vi "WT333.vi"(7 "simulazione":bool, 8 "error in (no error)":errorcluster, 11 "Queue Name":string="WT1600_Q") -> (0 "error out":errorcluster, 2 "Stopped":bool)   [LabVIEW 2019]
uses:
  TypeDef/MISURE WT.ctl
  TypeDef/DEVICE NAME.ctl
  <vilib>/Utility/file.llb/Read From Spreadsheet File (string).vi
  <vilib>/Utility/file.llb/Read Delimited Spreadsheet (string).vi
  <instrlib>/Yokogawa WT300 Series/Public/Data/Read Measurement (Normal).vi
  <instrlib>/Yokogawa WT300 Series/Yokogawa WT300 Series.lvlib
panel:
  out "length":i32
  out "read buffer 2":string
  out "Is Remote?":bool
  out "Is lockout?":bool
  in  "IS  REMOTE?":bool
  out "read buffer":string
  in  "IS LOCKOUT ?":bool
  in  "DIRETTO WT":bool
  in  "LEM 300":bool
  in  "LEM 1000":bool
  in  "LEM GENERICO":bool
  in  "write buffer":string=":INP:CURR:AUTO OFF;:INP:CURR:RANG EXT,1.0;"
  in  "CT Ratio (1.000)":dbl=0.2 format="%#_13g"
  out "Function":string[](array[string])
  out "WT330 Configuration":string[][](array[string])
  out "VISA resource name":refnum<visa-resource-name>
  in  "CONFIGURE":bool
  in  "SCELTA BANCO 2":bool
  out "Iteration":i32
  out "Measure":dbl[](array[numeric])
  out "MISURE WT":T1
  out "STATO":string
  out "LOOP TIME (ms)":u32
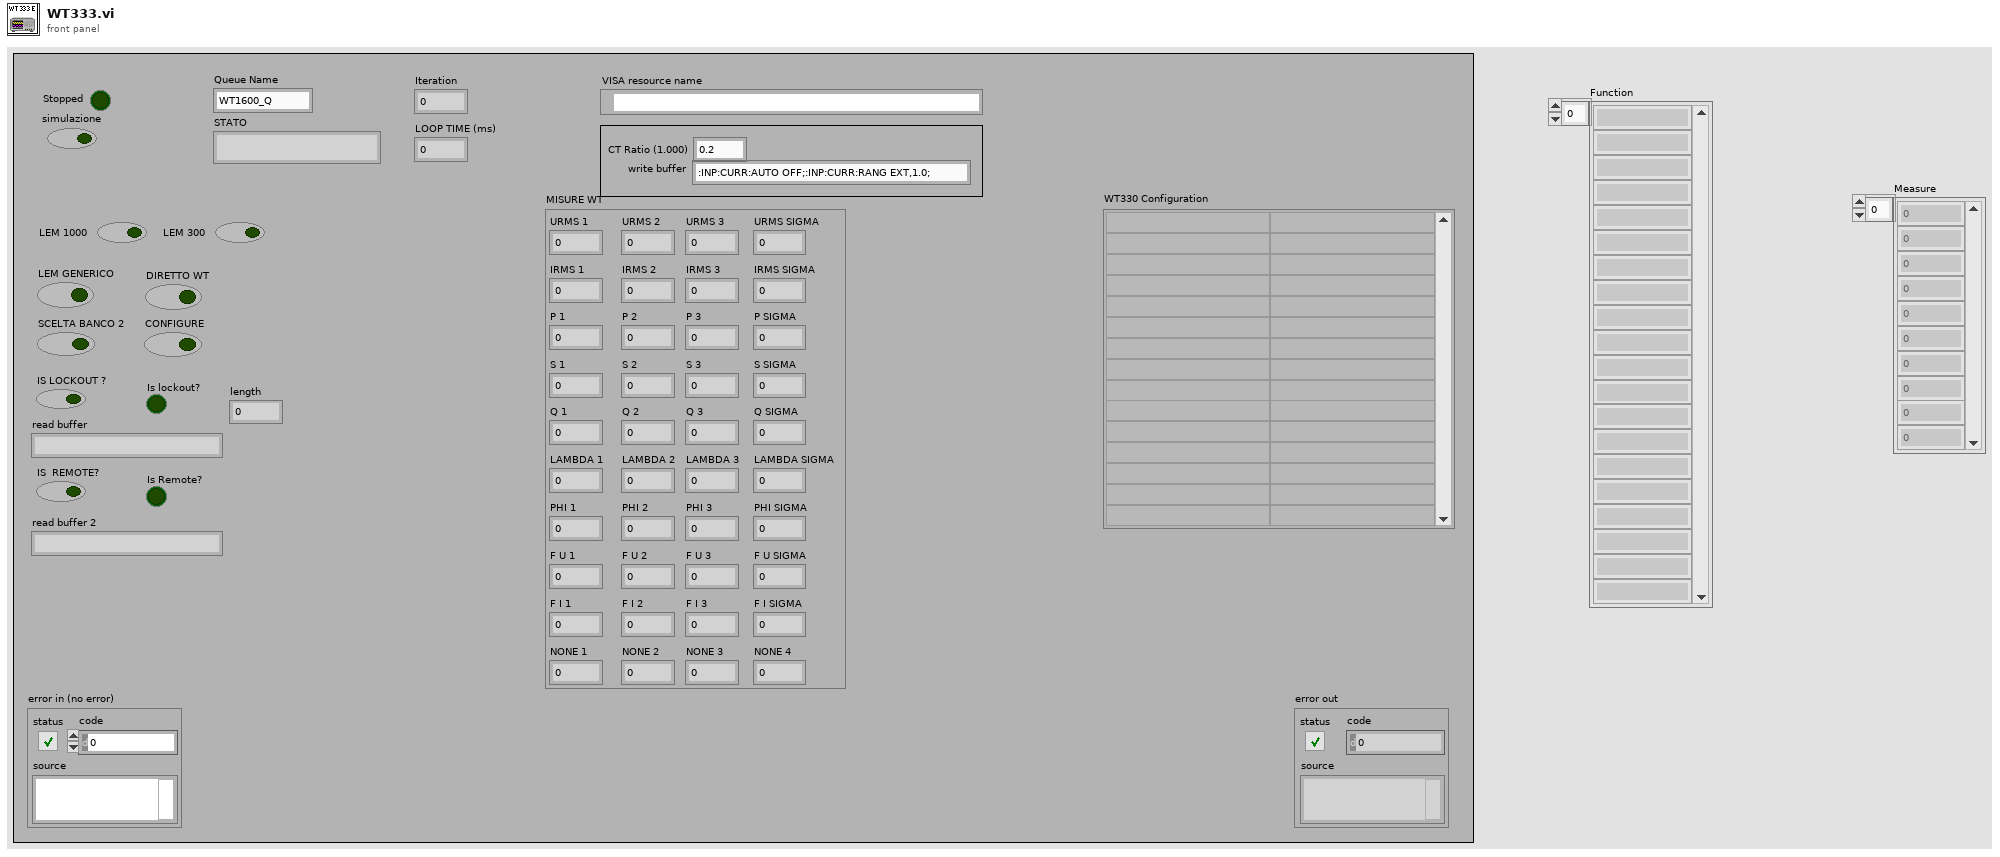
[diagram p1: front panel]
types:
  T1 = typedef "MISURE WT.ctl" = cluster{"URMS 1":dbl, "IRMS 1":dbl, "P 1":dbl, "S 1":dbl, "Q 1":dbl, "LAMBDA 1":dbl, "PHI 1":dbl, "F U 1":dbl, "F I 1":dbl, "NONE 1":dbl, "URMS 2":dbl, "IRMS 2":dbl, "P 2":dbl, "S 2":dbl, "Q 2":dbl, "LAMBDA 2":dbl, "PHI 2":dbl, "F U 2":dbl, "F I 2":dbl, "NONE 2":dbl, "URMS 3":dbl, "IRMS 3":dbl, "P 3":dbl, "S 3":dbl, "Q 3":dbl, "LAMBDA 3":dbl, "PHI 3":dbl, "F U 3":dbl, "F I 3":dbl, "NONE 3":dbl, "URMS SIGMA":dbl, "IRMS SIGMA":dbl, "P SIGMA":dbl, "S SIGMA":dbl, "Q SIGMA":dbl, "LAMBDA SIGMA":dbl, "PHI SIGMA":dbl, "F U SIGMA":dbl, "F I SIGMA":dbl, "NONE 4":dbl}
  T2 = typedef "DEVICE NAME.ctl" = enum16{"WATTMETRO", "APLUS", "PLC BANCO 1", "PLC RACK", "PLC BANCO 2", "PS", "NI cDAQ", "RESISTOMAT"}
  T3 = cluster{"Array of elements":cluster{"String":string, "variant":variant}[], "Single element":cluster{"String":string, "variant":variant}, "enque at\nopposite end (F)":bool, "no replications (F)":bool}
  T4 = cluster{"Measurement[0]":dbl, "Measurement[1]":dbl, "Measurement[2]":dbl, "Measurement[3]":dbl, "Measurement[4]":dbl, "Measurement[5]":dbl, "Measurement[6]":dbl, "Measurement[7]":dbl, "Measurement[8]":dbl, "Measurement[9]":dbl, "Measurement[10]":dbl, "Measurement[11]":dbl, "Measurement[12]":dbl, "Measurement[13]":dbl, "Measurement[14]":dbl, "Measurement[15]":dbl, "Measurement[16]":dbl, "Measurement[17]":dbl, "Measurement[18]":dbl, "Measurement[19]":dbl, "Measurement[20]":dbl, "Measurement[21]":dbl, "Measurement[22]":dbl, "Measurement[23]":dbl, "Measurement[24]":dbl, "Measurement[25]":dbl, "Measurement[26]":dbl, "Measurement[27]":dbl, "Measurement[28]":dbl, "Measurement[29]":dbl, "Measurement[30]":dbl, "Measurement[31]":dbl, "Measurement[32]":dbl, "Measurement[33]":dbl, "Measurement[34]":dbl, "Measurement[35]":dbl, "Measurement[36]":dbl, "Measurement[37]":dbl, "Measurement[38]":dbl, "Measurement[39]":dbl}
  T5 = enum32{"Invalid", "Standard", "Closed", "Hidden", "Minimized", "Maximized"}
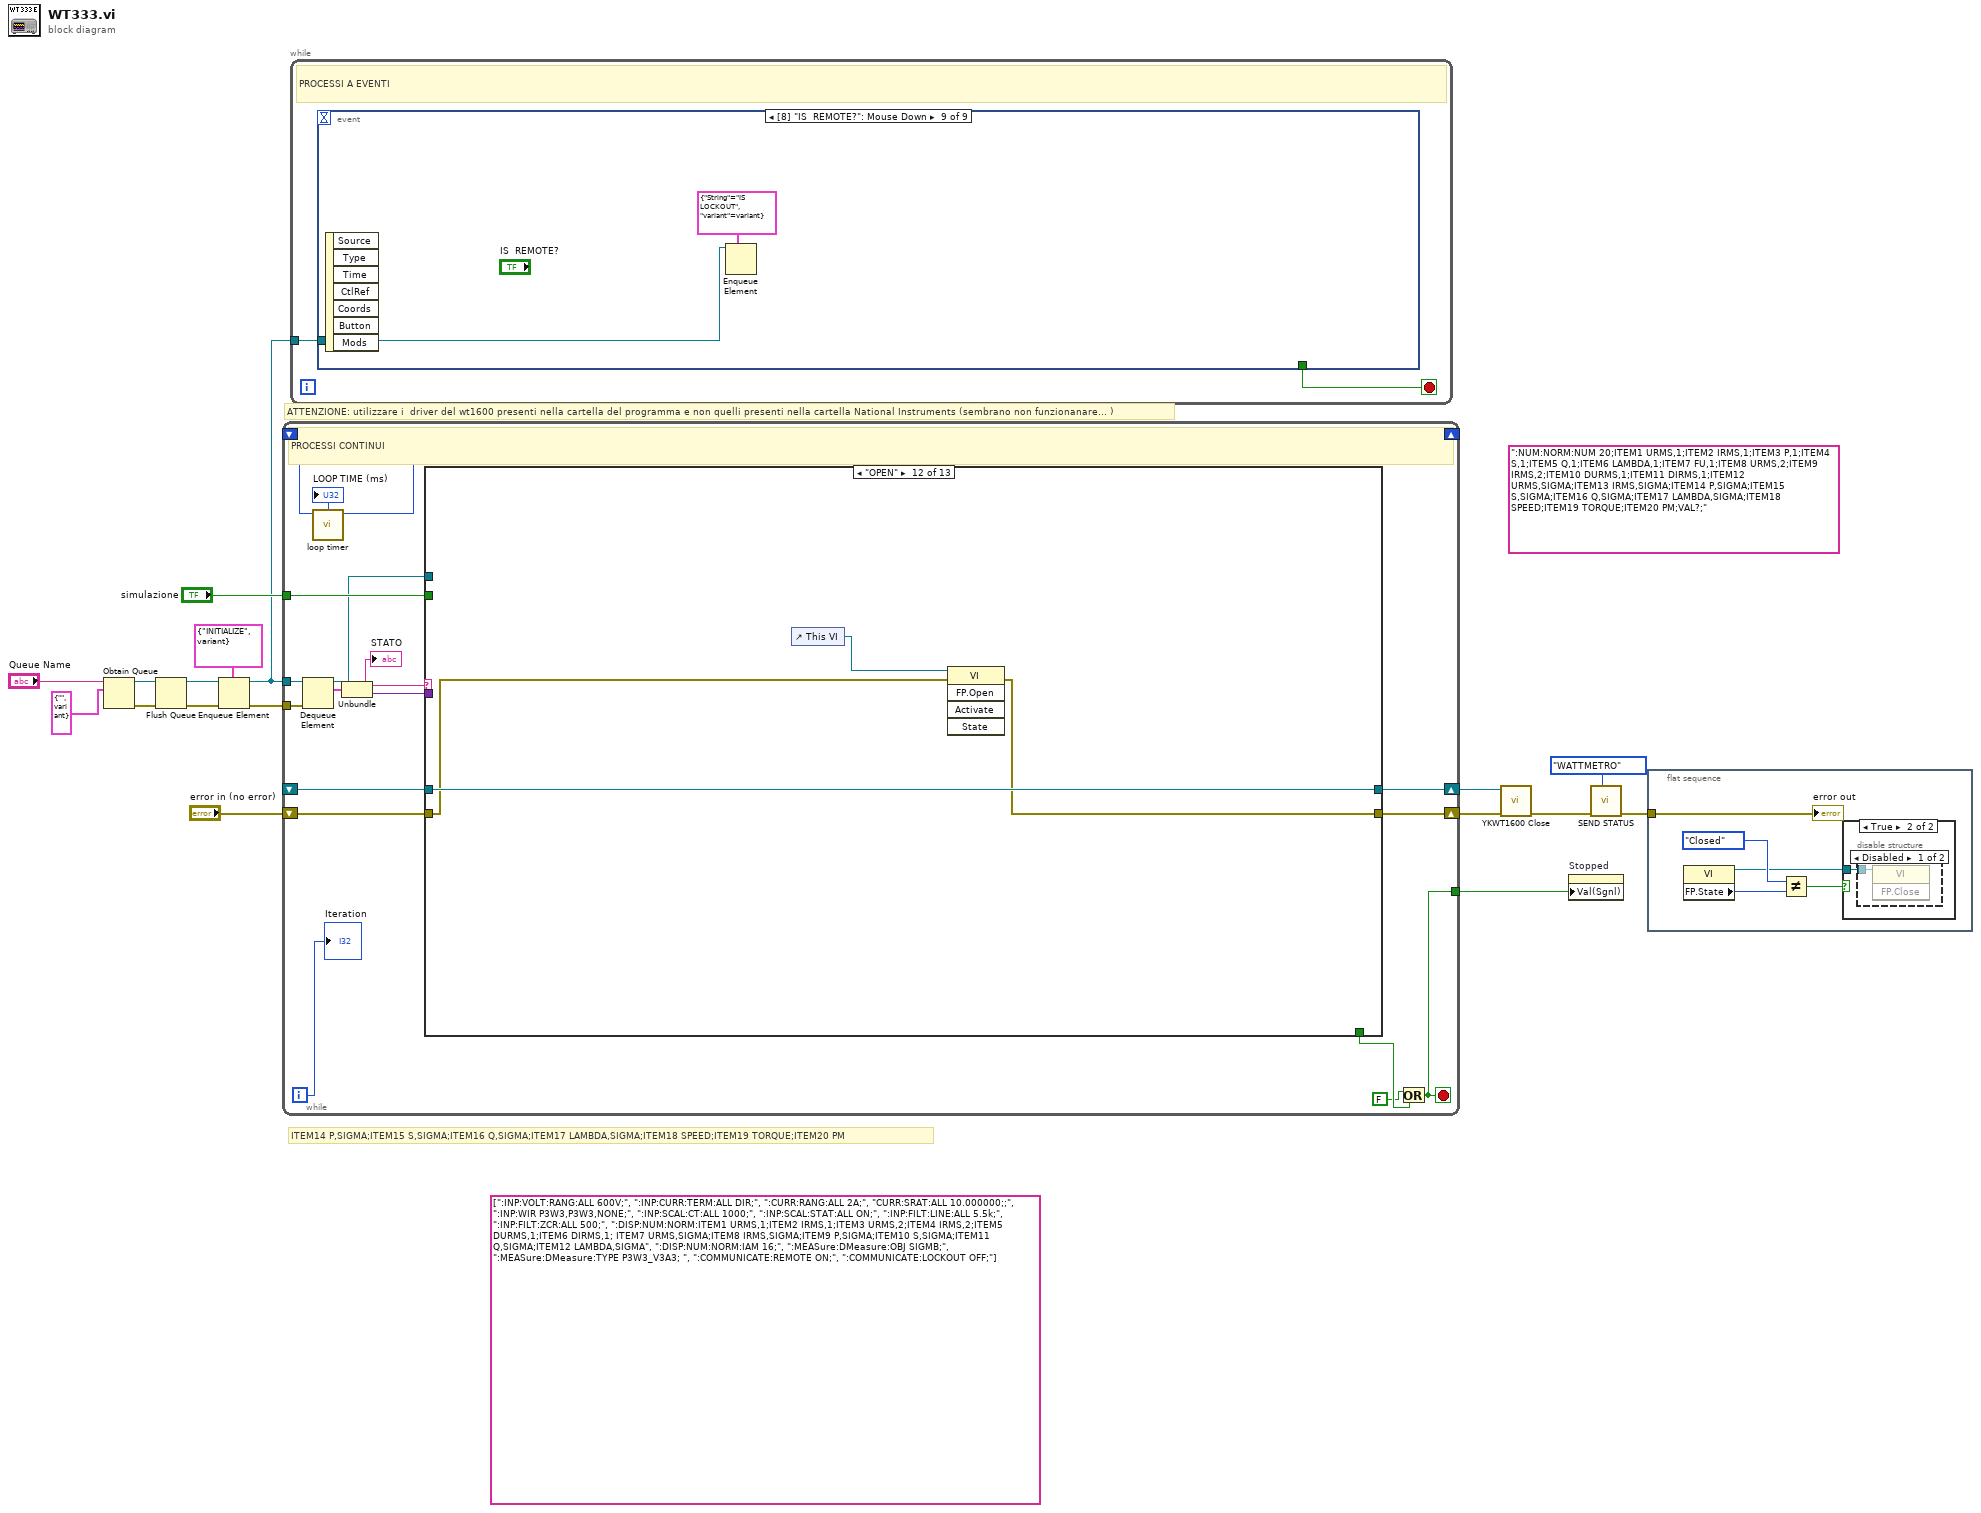
[diagram p0: block diagram]
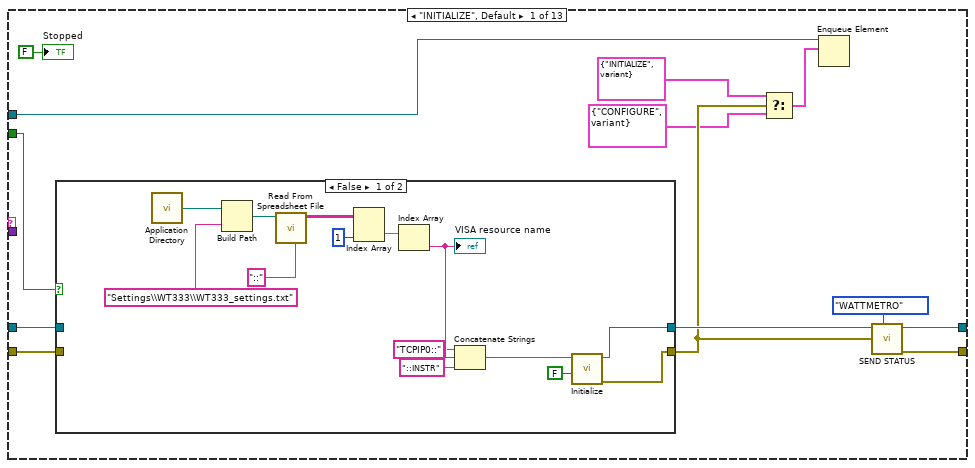
[diagram p2: hidden frame]
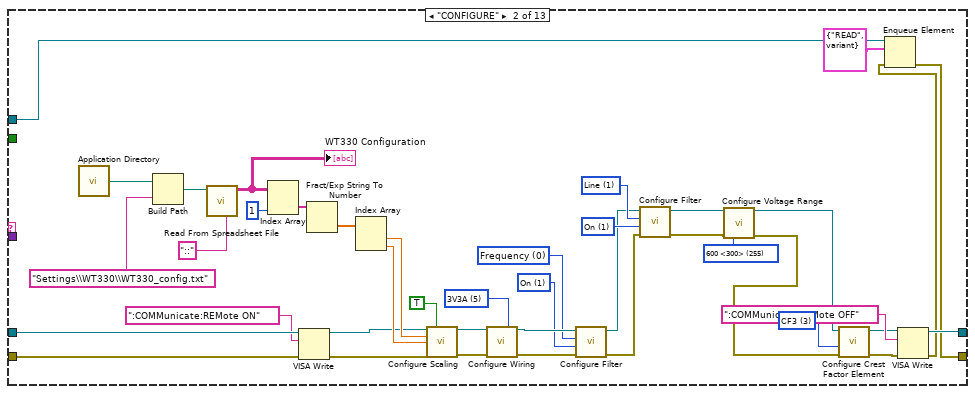
[diagram p4: hidden frame]
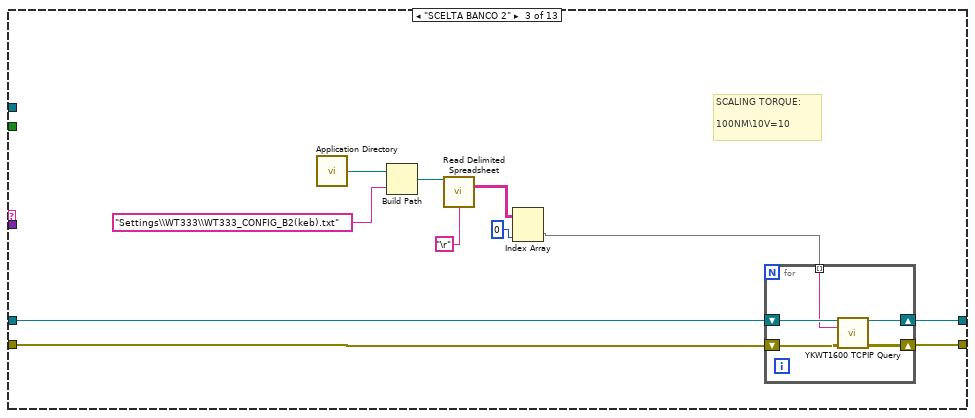
[diagram p5: hidden frame]
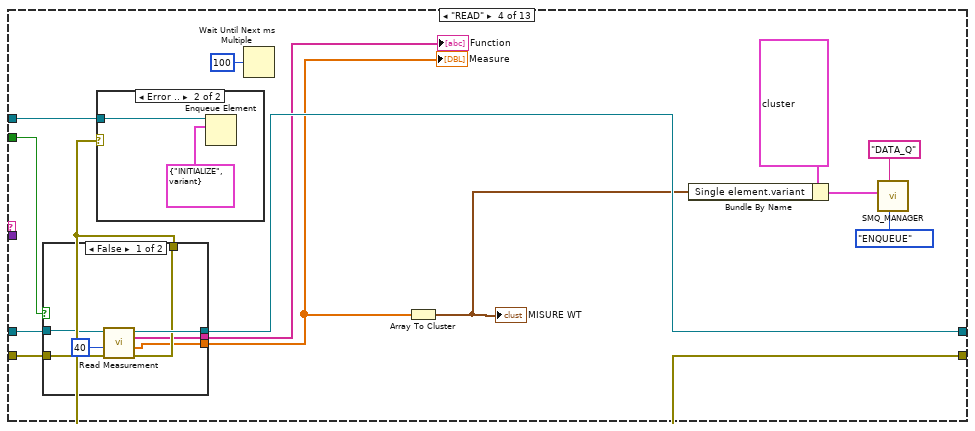
[diagram p6: hidden frame]
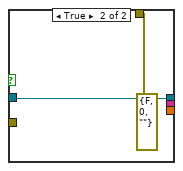
[diagram p7: hidden frame]
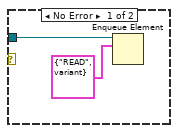
[diagram p8: hidden frame]
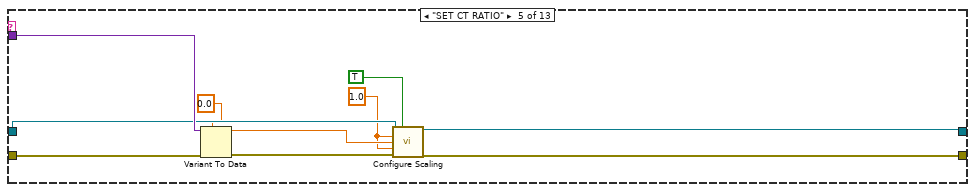
[diagram p9: hidden frame]
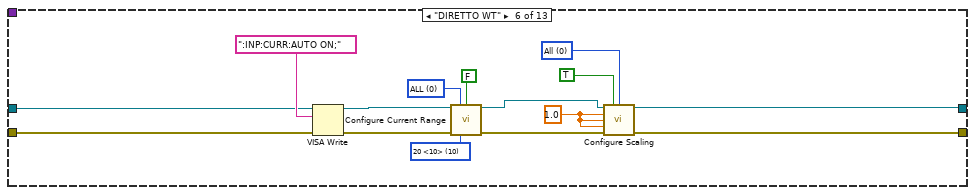
[diagram p10: hidden frame]
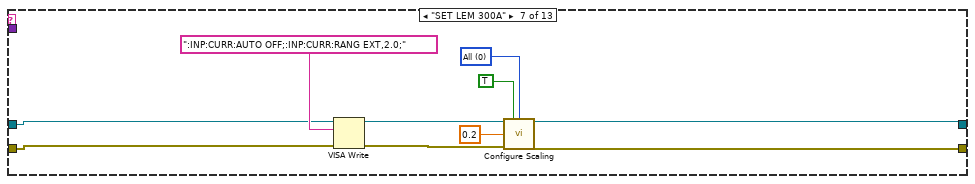
[diagram p11: hidden frame]
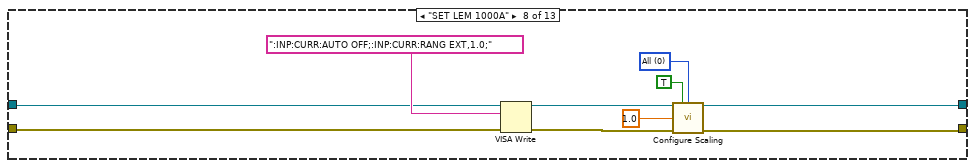
[diagram p12: hidden frame]
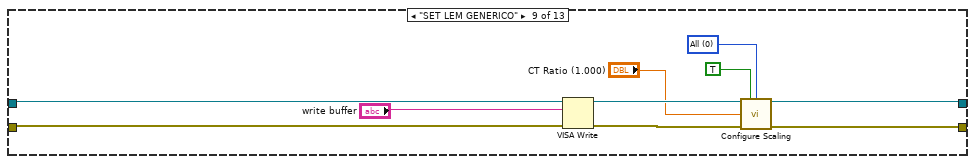
[diagram p13: hidden frame]
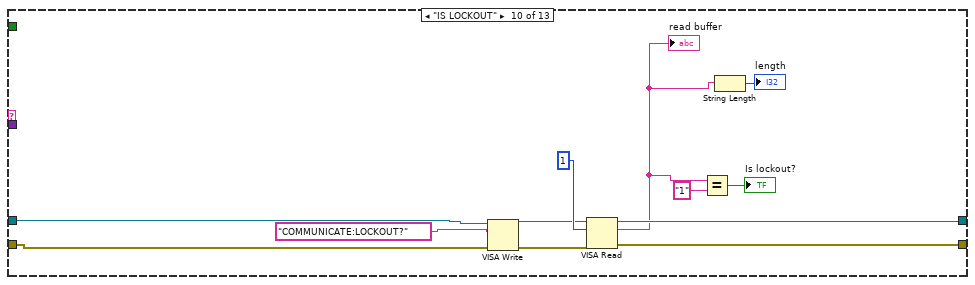
[diagram p14: hidden frame]
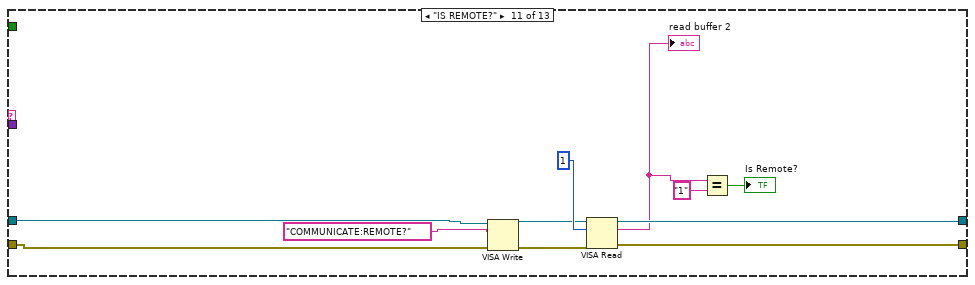
[diagram p15: hidden frame]
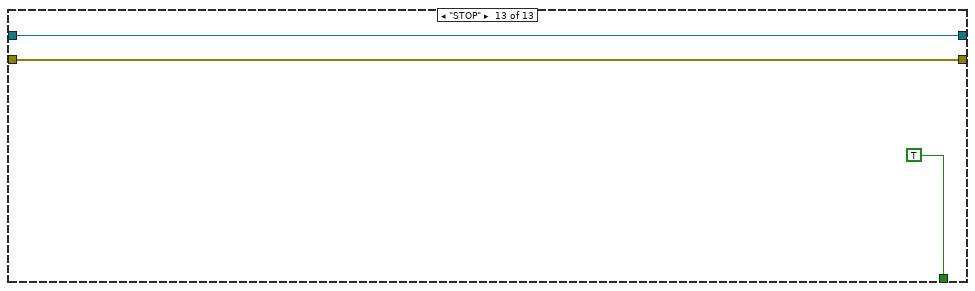
[diagram p16: hidden frame]
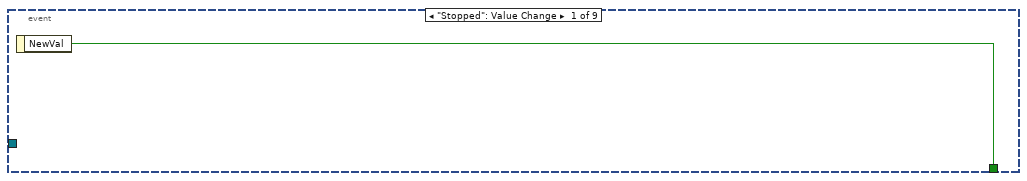
[diagram p19: hidden frame]
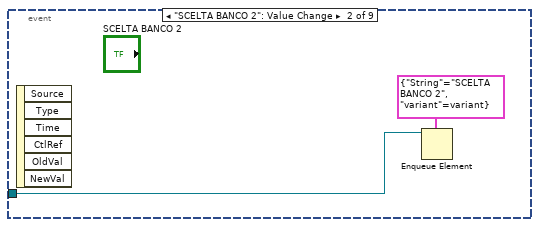
[diagram p20: hidden frame]
diagram:
  (unwired) string[] [":INP:VOLT:RANG:ALL 600V;", ":INP:CURR:TERM:ALL DIR;", ":CURR:RANG:ALL 2A;", "CURR:SRAT:ALL 10.000000;;", ":INP:WIR P3W3,P3W3,NONE;", ":INP:SCAL:CT:ALL 1000;", ":INP:SCAL:STAT:ALL ON;", ":INP:FILT:LINE:ALL 5.5k;", ":INP:FILT:ZCR:ALL 500;", ":DISP:NUM:NORM:ITEM1 URMS,1;ITEM2 IRMS,1;ITEM3 URMS,2;ITEM4 IRMS,2;ITEM5 DURMS,1;ITEM6 DIRMS,1; ITEM7 URMS,SIGMA;ITEM8 IRMS,SIGMA;ITEM9 P,SIGMA;ITEM10 S,SIGMA;ITEM11 Q,SIGMA;ITEM12 LAMBDA,SIGMA", ":DISP:NUM:NORM:IAM 16;", ":MEASure:DMeasure:OBJ SIGMB;", ":MEASure:DMeasure:TYPE P3W3_V3A3; ", ":COMMUNICATE:REMOTE ON;", ":COMMUNICATE:LOCKOUT OFF;"]
  (unwired) ":NUM:NORM:NUM 20;ITEM1 URMS,1;ITEM2 IRMS,1;ITEM3 P,1;ITEM4 S,1;ITEM5 Q,1;ITEM6 LAMBDA,1;ITEM7 FU,1;ITEM8 URMS,2;ITEM9 IRMS,2;ITEM10 DURMS,1;ITEM11 DIRMS,1;ITEM12 URMS,SIGMA;ITEM13 IRMS,SIGMA;ITEM14 P,SIGMA;ITEM15 S,SIGMA;ITEM16 Q,SIGMA;ITEM17 LAMBDA,SIGMA;ITEM18 SPEED;ITEM19 TORQUE;ITEM20 PM;VAL?;"
  # "CURR:SRAT:ALL 10.000000;"
  # "CURR:RANG:ALL 200MA"
  # "INP:CURR:TERM:ALL DIR"
  # "INP:VOLT:RANG:ALL 600V;"
  # "ITEM14 P,SIGMA;ITEM15 S,SIGMA;ITEM16 Q,SIGMA;ITEM17 LAMBDA,SIGMA;ITEM18 SPEED;ITEM19 TORQUE;ITEM20 PM"
  # "ATTENZIONE: utilizzare i  driver del wt1600 presenti nella cartella del programma e non quelli presenti nella cartella National Instruments (sembrano non funzionanare... )"
  n1 = Obtain Queue(name (unnamed)="Queue Name", element data type=cluster{"String":string, "variant":variant} {"String"="", "variant"=variant} ("element")) -> (queue out=w9:refnum<queue>, error out=w8:errorcluster)  [unwired: 3 in, 1 out]
  n2 = Flush Queue(queue=w9, error in (no error)=w8) -> (queue out=w7:refnum<queue>, error out=w6:errorcluster)  [unwired: 1 out]
  n3 = Enqueue Element(queue=w7, element=cluster{"String":string, "variant":variant} {"String"="INITIALIZE", "variant"=variant}, error in (no error)=w6) -> (queue out=w1:refnum<queue>, error out=w13:errorcluster)  [unwired: 1 in, 1 out]
  n4 = while {
    shift-right: [w35] -> _
    shift-left: _ -> [w34]
    shift-right: [w30] -> w4
    shift-left: "error in (no error)" -> [w32]
    tunnel: w1 -> [w28]
    tunnel: w13 -> [w29]
    tunnel: [w24] -> w14
    tunnel: "simulazione" -> [w23]
    shift-right: [w22] -> w5
    shift-left: _ -> [w21]
    i -> [w19]
    stop <- w24 stop-if-true
    # "PROCESSI CONTINUI"
    n5 = Dequeue Element(queue=w28, error in (no error)=w29) -> (queue out=w20:refnum<queue>, element=w27:cluster{"String":string, "variant":variant})  [unwired: 1 in, 2 out]
    n6 = call <userlib>:"loop timer.vi"("millisecond timer IN"=w34) -> ("millisecond timer OUT"=w35:u32, "LOOP TIME (ms)"=→"LOOP TIME (ms)":u32)  [unwired: 9 in]
    n7 = Unbundle(w27) -> ("String"=w26:string, "variant"=w25:variant)
    "STATO" <- w26
    n8 = case shown="\"OPEN\"" w26 {
      tunnel: [_ _ _ _ _ _ _ _ _ _ _ _ TRUE] -> w31
      tunnel: w32 -> [w46 w71 w115 w132 w156 w162 w176 w183 w195 w214 w225 w228 w231]
      tunnel: [w40 w64 w114 w126 w148 w158 w173 w185 w193 w207 w218 w227 w231] -> w30
      tunnel: w25 -> [_ _ _ _ w155 _ _ _ _ _ _ _ _]
      tunnel: w23 -> [w45 _ _ w124 _ _ _ _ _ _ _ _ _]
      tunnel: [w43 w67 w112 w131 w149 w159 w174 w186 w194 w208 w219 w229 w230] -> w22
      tunnel: w21 -> [w44 w74 w113 w127 w154 w163 w175 w184 w196 w213 w224 w229 w230]
      tunnel: w20 -> [w42 w104 _ w125 _ _ _ _ _ _ _ _ _]
      frame "INITIALIZE", Default {
        n9 = case shown="False" w45 {
          tunnel: w46 -> [_ w63]
          tunnel: [w48 w63] -> w39
          tunnel: [w49 w62] -> w43
          tunnel: w44 -> [_ w62]
          frame False {
            n10 = call <vilib>:"Application Directory.vi"() -> ("Application Directory"=w55:path)
            n11 = Build Path(base path=w55, name or relative path="Settings\\WT333\\WT333_settings.txt") -> (appended path=w57:path)
            n12 = call-poly <vilib>:"Read From Spreadsheet File.vi"("delimiter (\\t)"="::" ("delimiter (\\t)"), "file path (dialog if empty)"=w57) -> ("all rows"=w59:string[][])  [unwired: 5 in, 4 out]
            n13 = Index Array(array=w59, index (col)=1 ("disabled index (col)")) -> (element=w61:string[])  [unwired: 1 in]
            n14 = Index Array(array=w61) -> (element=w52:string)  [unwired: 1 in]
            "VISA resource name" <- w52
            n15 = Concatenate Strings("TCPIP0::" ("string"), w52, "::INSTR" ("string")) -> (w53:string)
            n16 = call <instrlib>:"Initialize.vi"("Reset (True)"=FALSE, "VISA resource name"=w53) -> ("error out"=w48:errorcluster, "VISA resource name out"=w49:refnum<visa-resource-name>)  [unwired: 8 in]
          }
          frame True {
          }
        }
        n17 = Select(t=cluster{"String":string, "variant":variant} {"String"="INITIALIZE", "variant"=variant} ("element"), s=w39, f=cluster{"String":string, "variant":variant} {"String"="CONFIGURE", "variant"=variant} ("element")) -> (s? t:f=w38:cluster{"String":string, "variant":variant})
        n18 = Enqueue Element(queue=w42, element=w38) -> ()  [unwired: 2 in, 3 out]
        n19 = call "SEND STATUS.vi"("ELEMENT"=DEVICE_NAME."WATTMETRO", "error in (no error)"=w39) -> ("error out"=w40:errorcluster)  [unwired: 9 in]
        "Stopped" <- FALSE ("Stop")
      }
      frame "CONFIGURE" {
        w98 = u8 255 items=["15 <7.5>"=8, "30 <15>"=15, "60 <30>"=30, "150 <75>"=75, "300 <150>"=150, "600 <300>"=255] ("Manual Range (600 <300> V)")
        w97 = 1 items=["Off", "On"] ("Set Filter (1: On)")
        w96 = u32 1 items=["Frequency", "Line"] ("Select Filter Type (0 : Frequency)")
        w92 = 3 items=["CF3"=3, "CF6"=6] ("Crest Factor (3: CF3)")
        w91 = 5 items=["1P2W"=1, "1P3W"=2, "3P3W"=3, "3P4W"=4, "3V3A"=5] ("Wiring A (1: 1p2W)")
        w86 = 1 items=["Off", "On"] ("Set Filter (1: On)")
        w85 = u32 0 items=["Frequency", "Line"] ("Select Filter Type (0 : Frequency)")
        n20 = call <vilib>:"Application Directory.vi"() -> ("Application Directory"=w76:path)
        n21 = Build Path(base path=w76, name or relative path="Settings\\WT330\\WT330_config.txt") -> (appended path=w78:path)
        n22 = call-poly <vilib>:"Read From Spreadsheet File.vi"("delimiter (\\t)"="::" ("delimiter (\\t)"), "file path (dialog if empty)"=w78) -> ("all rows"=w80:string[][])  [unwired: 5 in, 4 out]
        "WT330 Configuration" <- w80
        n23 = Index Array(array=w80, index (col)=1 ("disabled index (col)")) -> (element=w82:string[])  [unwired: 1 in]
        n24 = VISA Write ("VISA書き込み")(VISA resource name=w74, write buffer=":COMMunicate:REMote ON", error in (no error)=w71) -> (VISA resource name out=w73:refnum<visa-resource-name>, error out=w70:errorcluster)  [unwired: 1 out]
        n25 = Fract/Exp String To Number(string=w82) -> (number=w83:dbl[])  [unwired: 3 in, 1 out]
        n26 = Index Array(array=w83) -> (element #1=w93:dbl, element #2=w84:dbl)  [unwired: 2 in]
        n27 = call <instrlib>:"Configure Scaling.vi"("VISA resource name"=w73, "Enable Scaling (T: Enable)"=TRUE, "VT Ratio (1.000)"=w93, "CT Ratio (1.000)"=w84, "error in (no error)"=w70) -> ("VISA resource name out"=w87:refnum<visa-resource-name>, "error out"=w88:errorcluster)  [unwired: 9 in]
        n28 = call <instrlib>:"Configure Wiring.vi"("VISA resource name"=w87, "Wiring A (1: 1p2W)"=w91, "error in (no error)"=w88) -> ("VISA resource name out"=w89:refnum<visa-resource-name>, "error out"=w90:errorcluster)  [unwired: 11 in]
        n29 = call <instrlib>:"Configure Filter.vi"("error in (no error)"=w90, "Set Filter (1: On)"=w86, "Select Filter Type (0 : Frequency)"=w85, "VISA resource name"=w89) -> ("error out"=w95:errorcluster, "VISA resource name out"=w94:refnum<visa-resource-name>)  [unwired: 6 in]
        n30 = call <instrlib>:"Configure Filter.vi"("error in (no error)"=w95, "Set Filter (1: On)"=w97, "Select Filter Type (0 : Frequency)"=w96, "VISA resource name"=w94) -> ("error out"=w101:errorcluster, "VISA resource name out"=w99:refnum<visa-resource-name>)  [unwired: 6 in]
        n31 = call <instrlib>:"Configure Voltage Range.vi"("VISA resource name"=w99, "error in (no error)"=w101, "Manual Range (600 <300> V)"=w98) -> ("VISA resource name out"=w100:refnum<visa-resource-name>, "error out"=w102:errorcluster)  [unwired: 11 in]
        n32 = call <instrlib>:"Configure Crest Factor Element.vi"("error in (no error)"=w102, "Crest Factor (3: CF3)"=w92, "VISA resource name"=w100) -> ("error out"=w66:errorcluster, "VISA resource name out"=w68:refnum<visa-resource-name>)  [unwired: 7 in]
        n33 = VISA Write ("VISA書き込み")(VISA resource name=w68, write buffer=":COMMunicate:REMote OFF", error in (no error)=w66) -> (VISA resource name out=w67:refnum<visa-resource-name>, error out=w65:errorcluster)  [unwired: 1 out]
        n34 = Enqueue Element(queue=w104, element=cluster{"String":string, "variant":variant} {"String"="READ", "variant"=variant}, error in (no error)=w65) -> (error out=w64:errorcluster)  [unwired: 1 in, 2 out]
      }
      frame "SCELTA BANCO 2" {
        # "SCALING TORQUE:\n\n100NM\\10V=10"
        n35 = call <vilib>:"Application Directory.vi"() -> ("Application Directory"=w111:path)
        n36 = Build Path(base path=w111, name or relative path="Settings\\WT333\\WT333_CONFIG_B2(keb).txt") -> (appended path=w110:path)
        n37 = call-poly <vilib>:"Read Delimited Spreadsheet.vi"("file path (dialog if empty)"=w110, "delimiter (\\t)"="\r") -> ("all rows"=w109:string[][])  [unwired: 8 in, 5 out]
        n38 = Index Array(array=w109, index (col)=0 ("index (row)")) -> (element=w105:string[])  [unwired: 1 in]
        n39 = for {
          tunnel: w105 -> [w116] mode=indexing
          shift-right: [w119] -> w114
          shift-left: w115 -> [w120]
          shift-right: [w117] -> w112
          shift-left: w113 -> [w118]
          n40 = call "YKWT1600 TCPIP Query.vi"("VISA session"=w118, "Write Data"=w116, "error in (no error)"=w120) -> ("dup VISA session"=w117:refnum<visa-resource-name>, "error out"=w119:errorcluster)  [unwired: 9 in, 2 out]
        }
      }
      frame "READ" {
        n41 = case shown="False" w124 {
          tunnel: w132 -> [w141 _]
          tunnel: [w139 w143] -> w131
          tunnel: [w136 _] -> w123
          tunnel: w127 -> [w140 w143]
          tunnel: [w137 _] -> w122
          tunnel: [w138 errorcluster {"status"=FALSE, "code"=0, "source"=""} ("error out")] -> w126
          frame False {
            n42 = call-poly <instrlib>:"Read Measurement.vi"("error in (no error)"=w141, "Number of Item (15)"=40, "VISA resource name"=w140) -> ("error out"=w138:errorcluster, "Measurement"=w137:dbl[], "Function"=w136:string[], "VISA resource name out"=w139:refnum<visa-resource-name>)  [unwired: 5 in]
          }
          frame True {
          }
        }
        "Measure" <- w122
        "Function" <- w123
        n43 = case shown="Error .." w126 {
          tunnel: w125 -> [w145 w146]
          frame No Error {
            n44 = Enqueue Element(queue=w145, element=cluster{"String":string, "variant":variant} {"String"="READ", "variant"=variant}) -> ()  [unwired: 2 in, 3 out]
          }
          frame Error {
            n45 = Enqueue Element(queue=w146, element=cluster{"String":string, "variant":variant} {"String"="INITIALIZE", "variant"=variant}) -> ()  [unwired: 2 in, 3 out]
          }
        }
        n46 = Wait Until Next ms Multiple(millisecond multiple=u32 100) -> ()  [unwired: 1 out]
        n47 = Array To Cluster(array=w122) -> (cluster=w121:T4)
        "MISURE WT" <- w121
        n48 = Bundle By Name(cluster=T3 {"Array of elements"=[], "Single element"={"String"="READ WT", "variant"=variant}, "enque at\nopposite end (F)"=FALSE, "no replications (F)"=FALSE} ("Enqueue cluster"), "Single element.variant"=w121) -> (w133:T3)
        n49 = call <userlib>:"SMQ_MANAGER.vi"("Function"=enum16{"INITIALIZE", "ENQUEUE", "STOP ALL"}."ENQUEUE", "Queue name"="DATA_Q", "Enqueue cluster"=w133) -> ()  [unwired: 8 in, 1 out]
      }
      frame "SET CT RATIO" {
        w151 = 1.0 ("VT Ratio (1.000)")
        n50 = Variant To Data(error in=w156, type=0.0, Variant=w155) -> (data=w152:dbl, error out=w157:errorcluster)
        n51 = call <instrlib>:"Configure Scaling.vi"("VISA resource name"=w154, "Enable Scaling (T: Enable)"=TRUE, "VT Ratio (1.000)"=w151, "CT Ratio (1.000)"=w152, "Power Coefficient (1.000)"=w151, "error in (no error)"=w157) -> ("VISA resource name out"=w149:refnum<visa-resource-name>, "error out"=w148:errorcluster)  [unwired: 8 in]
      }
      frame "DIRETTO WT" {
        w172 = u8 10 items=["5m <2.5m>"=0, "10m <5m>"=0, "20m <10m>"=0, "50m <25m>"=0, "100m <50m>"=0, "200m <100m>"=0, "500m <250m>"=0, "1 <500m>"=0, "2 <1>"=1, "5 <2.5>"=2, "10 <5>"=5, "20 <10>"=10, "40 <20>"=20] ("Manual Range (20 <10> A)")
        w171 = u8 0 items=["ALL", "Custom"] ("Range Type (1: Custom)")
        w167 = 1.0 ("VT Ratio (1.000)")
        w164 = 0 items=["All", "1", "2", "3"] ("Element (0: All)")
        n52 = VISA Write ("VISA書き込み")(VISA resource name=w163, write buffer=":INP:CURR:AUTO ON;", error in (no error)=w162) -> (VISA resource name out=w168:refnum<visa-resource-name>, error out=w161:errorcluster)  [unwired: 1 out]
        n53 = call <instrlib>:"Configure Current Range.vi"("VISA resource name"=w168, "Range Type (1: Custom)"=w171, "Enable Auto Range (F: Disable)"=FALSE, "error in (no error)"=w161, "Manual Range (20 <10> A)"=w172) -> ("VISA resource name out"=w169:refnum<visa-resource-name>, "error out"=w160:errorcluster)  [unwired: 9 in]
        n54 = call <instrlib>:"Configure Scaling.vi"("VISA resource name"=w169, "Enable Scaling (T: Enable)"=TRUE, "Element (0: All)"=w164, "VT Ratio (1.000)"=w167, "CT Ratio (1.000)"=w167, "Power Coefficient (1.000)"=w167, "error in (no error)"=w160) -> ("VISA resource name out"=w159:refnum<visa-resource-name>, "error out"=w158:errorcluster)  [unwired: 7 in]
      }
      frame "SET LEM 300A" {
        w177 = 0 items=["All", "1", "2", "3"] ("Element (0: All)")
        n55 = VISA Write ("VISA書き込み")(VISA resource name=w175, write buffer=":INP:CURR:AUTO OFF;:INP:CURR:RANG EXT,2.0;", error in (no error)=w176) -> (VISA resource name out=w179:refnum<visa-resource-name>, error out=w180:errorcluster)  [unwired: 1 out]
        n56 = call <instrlib>:"Configure Scaling.vi"("VISA resource name"=w179, "Enable Scaling (T: Enable)"=TRUE, "Element (0: All)"=w177, "CT Ratio (1.000)"=0.2, "error in (no error)"=w180) -> ("VISA resource name out"=w174:refnum<visa-resource-name>, "error out"=w173:errorcluster)  [unwired: 9 in]
      }
      frame "SET LEM 1000A" {
        w189 = 0 items=["All", "1", "2", "3"] ("Element (0: All)")
        n57 = VISA Write ("VISA書き込み")(VISA resource name=w184, write buffer=":INP:CURR:AUTO OFF;:INP:CURR:RANG EXT,1.0;", error in (no error)=w183) -> (VISA resource name out=w190:refnum<visa-resource-name>, error out=w191:errorcluster)  [unwired: 1 out]
        n58 = call <instrlib>:"Configure Scaling.vi"("VISA resource name"=w190, "Enable Scaling (T: Enable)"=TRUE, "Element (0: All)"=w189, "CT Ratio (1.000)"=1.0, "error in (no error)"=w191) -> ("VISA resource name out"=w186:refnum<visa-resource-name>, "error out"=w185:errorcluster)  [unwired: 9 in]
      }
      frame "SET LEM GENERICO" {
        w197 = 0 items=["All", "1", "2", "3"] ("Element (0: All)")
        n59 = VISA Write ("VISA書き込み")(VISA resource name=w196, write buffer="write buffer", error in (no error)=w195) -> (VISA resource name out=w202:refnum<visa-resource-name>, error out=w199:errorcluster)  [unwired: 1 out]
        n60 = call <instrlib>:"Configure Scaling.vi"("VISA resource name"=w202, "Enable Scaling (T: Enable)"=TRUE, "Element (0: All)"=w197, "CT Ratio (1.000)"="CT Ratio (1.000)", "error in (no error)"=w199) -> ("VISA resource name out"=w194:refnum<visa-resource-name>, "error out"=w193:errorcluster)  [unwired: 9 in]
      }
      frame "IS LOCKOUT" {
        n61 = VISA Write(VISA resource name=w213, write buffer="COMMUNICATE:LOCKOUT?", error in (no error)=w214) -> (VISA resource name out=w210:refnum<visa-resource-name>, error out=w209:errorcluster)  [unwired: 1 out]
        n62 = VISA Read(VISA resource name=w210, byte count=u32 1, error in (no error)=w209) -> (VISA resource name out=w208:refnum<visa-resource-name>, read buffer=w204:string, error out=w207:errorcluster)  [unwired: 1 out]
        "read buffer" <- w204
        n63 = Equal?(x=w204, y="1") -> (x = y?=→"Is lockout?":bool)
        n64 = String Length(string=w204) -> (length=→"length":i32)
      }
      frame "IS REMOTE?" {
        n65 = VISA Write(VISA resource name=w224, write buffer="COMMUNICATE:REMOTE?", error in (no error)=w225) -> (VISA resource name out=w221:refnum<visa-resource-name>, error out=w220:errorcluster)  [unwired: 1 out]
        n66 = VISA Read(VISA resource name=w221, byte count=u32 1, error in (no error)=w220) -> (VISA resource name out=w219:refnum<visa-resource-name>, read buffer=w217:string, error out=w218:errorcluster)  [unwired: 1 out]
        "read buffer 2" <- w217
        n67 = Equal?(x=w217, y="1") -> (x = y?=→"Is Remote?":bool)
      }
      frame "OPEN" {
        n68 = control-ref of="This VI"() -> (w226:refnum<vi>)
        n69 = invoke class="VI" method="FP.Open"(reference=w226, error in=w228) -> (error out=w227:errorcluster)  [unwired: 3 in, 4 out]
      }
      frame "STOP" {
      }
    }
    n70 = Or(x=FALSE, y=w31) -> (x .or. y?=w24:bool)
    "Iteration" <- w19
  }
  n71 = while {
    tunnel: w1 -> [w233]
    stop <- w234 stop-if-true
    # "PROCESSI A EVENTI"
    n72 = event shown="[8] \"IS  REMOTE?\": Mouse Down" {
      selector: _ -> [_ _ _ _ _ _ _ _ _]
      dyn-events: _ -> [_ _ _ _ _ _ _ _ _]
      timeout: _ -> [_ _ _ _ _ _ _ _ _]
      tunnel: [w235 _ _ _ _ _ _ _ _] -> w234
      tunnel: w233 -> [_ w236 w238 w240 w242 w244 w246 w248 w250]
      event "Stopped": Value Change {
        n73 = event-data() -> ("NewVal"=w235:bool)  [unwired: 1 in]
      }
      event "SCELTA BANCO 2": Value Change {
        n74 = event-data() -> ()  [unwired: 1 in, 6 out]
        n75 = Enqueue Element(queue=w236, element=cluster{"String":string, "variant":variant} {"String"="SCELTA BANCO 2", "variant"=variant}) -> ()  [unwired: 2 in, 3 out]
      }
      event "CONFIGURE": Value Change {
        n76 = event-data() -> ()  [unwired: 1 in, 6 out]
        n77 = Enqueue Element(queue=w238, element=cluster{"String":string, "variant":variant} {"String"="CONFIGURE", "variant"=variant}) -> ()  [unwired: 2 in, 3 out]
      }
      event "LEM 300": Value Change {
        n78 = event-data() -> ()  [unwired: 1 in, 6 out]
        n79 = Enqueue Element(queue=w240, element=cluster{"String":string, "variant":variant} {"String"="SET LEM 300A", "variant"=variant}) -> ()  [unwired: 2 in, 3 out]
      }
      event "LEM 1000": Value Change {
        n80 = event-data() -> ()  [unwired: 1 in, 6 out]
        n81 = Enqueue Element(queue=w242, element=cluster{"String":string, "variant":variant} {"String"="SET LEM 1000A", "variant"=variant}) -> ()  [unwired: 2 in, 3 out]
      }
      event "LEM GENERICO": Value Change {
        n82 = event-data() -> ()  [unwired: 1 in, 6 out]
        n83 = Enqueue Element(queue=w244, element=cluster{"String":string, "variant":variant} {"String"="SET LEM GENERICO", "variant"=variant}) -> ()  [unwired: 2 in, 3 out]
      }
      event "DIRETTO WT": Value Change {
        n84 = event-data() -> ()  [unwired: 1 in, 6 out]
        n85 = Enqueue Element(queue=w246, element=cluster{"String":string, "variant":variant} {"String"="DIRETTO WT", "variant"=variant}) -> ()  [unwired: 2 in, 3 out]
      }
      event "IS LOCKOUT ?": Mouse Down {
        n86 = event-data() -> ()  [unwired: 1 in, 7 out]
        n87 = Enqueue Element(queue=w248, element=cluster{"String":string, "variant":variant} {"String"="IS LOCKOUT", "variant"=variant}) -> ()  [unwired: 2 in, 3 out]
      }
      event "IS  REMOTE?": Mouse Down {
        n88 = event-data() -> ()  [unwired: 1 in, 7 out]
        n89 = Enqueue Element(queue=w250, element=cluster{"String":string, "variant":variant} {"String"="IS LOCKOUT", "variant"=variant}) -> ()  [unwired: 2 in, 3 out]
      }
    }
  }
  n90 = call "YKWT1600 Close.vi"("VISA session"=w5, "error in (no error)"=w4) -> ("error out"=w3:errorcluster)  [unwired: 13 in]
  n91 = property on="Stopped" class="Bool (strict)"("Val(Sgnl)"=w14) -> ()  [unwired: 2 in, 2 out]
  n92 = call "SEND STATUS.vi"("ELEMENT"=DEVICE_NAME."WATTMETRO", "error in (no error)"=w3) -> ("error out"=w11:errorcluster)  [unwired: 9 in]
  n93 = flat-sequence {
    tunnel: w11 -> [w252]
    frame #0 {
      n94 = property class="VI"() -> (reference out=w253:refnum<vi>, "FP.State"=w256:T5)  [unwired: 2 in, 1 out]
      n95 = Not Equal?(x=T5."Closed", y=w256) -> (x != y?=w254:bool)
      n96 = case shown="True" w254 {
        tunnel: w253 -> [_ w257]
        frame False {
        }
        frame True {
          n97 = disable-structure shown="Disabled" {
            disable-tunnel: w257 -> [w258 _]
            frame Disabled {
              n98 = invoke class="VI" method="FP.Close"(reference=w258) -> ()  [unwired: 2 in, 3 out]
            }
            frame Enabled {
            }
          }
        }
      }
      "error out" <- w252
    }
  }
